vi "VI Scripting with Structures - Timed Loop.vi"   [LabVIEW 2023]
doc: "This example contains sample code demonstrating common VI Scripting navigational tasks relating to Timed Loops."
panel:
  # "Overview: Illustrates several TimedLoop properties and methods used for inspecting and modifying Timed Loops with VI Scripting.\nInstructions:\nOpen the block diagram of this VI to see several examples of properties and methods related to Timed Loops and VI Scripting.\n\nNote: Browse the diagram of this example to learn about VI Scripting concepts. This example is not meant to be run."
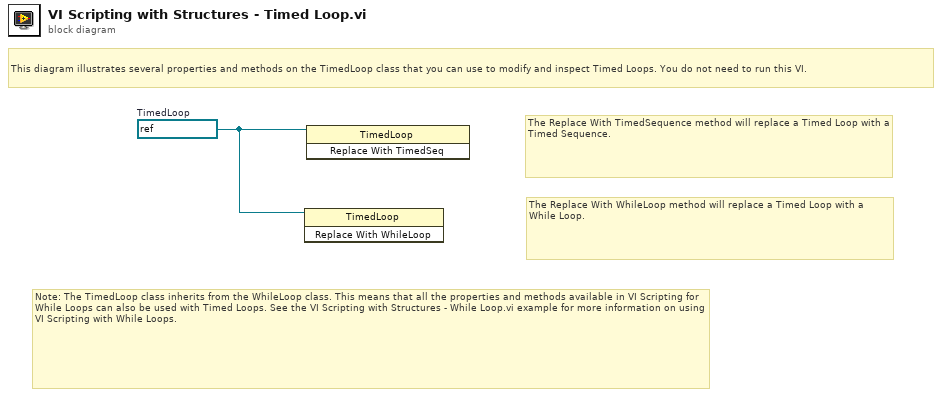
[diagram p0: block diagram]
diagram:
  w1 = refnum<vi> refnum  # TimedLoop
  # "Note: The TimedLoop class inherits from the WhileLoop class. This means that all the properties and methods available in VI Scripting for While Loops can also be used with Timed Loops. See the VI Scripting with Structures - While Loop.vi example for more information on using VI Scripting with While Loops."
  # "The Replace With WhileLoop method will replace a Timed Loop with a While Loop."
  # "The Replace With TimedSequence method will replace a Timed Loop with a Timed Sequence."
  # "This diagram illustrates several properties and methods on the TimedLoop class that you can use to modify and inspect Timed Loops. You do not need to run this VI."
  n1 = invoke class="TimedLoop" method="Replace With WhileLoop"(reference=w1) -> ()  [unwired: 2 in, 3 out]
  n2 = invoke class="TimedLoop" method="Replace With TimedSeq"(reference=w1) -> ()  [unwired: 2 in, 3 out]
